vi "get Object By Name.vi"(10 "Name":string, 11 "Scene in":refnum<class "Scene.lvclass">) -> (2 "Index":i32, 3 "Object":T1)   [LabVIEW 2022 SP3, in "Application.lvlib" / "Scene.lvclass"]
uses:
  Scene.lvclass
  Libraries/3D/Object.ctl
  Libraries/3D/Triangle 3D.ctl
  Libraries/3D/Vector 3D.ctl
  Libraries/3D/Transform.ctl
  Scene.lvclass/Scene.ctl
  Libraries/3D/3D.lvlib
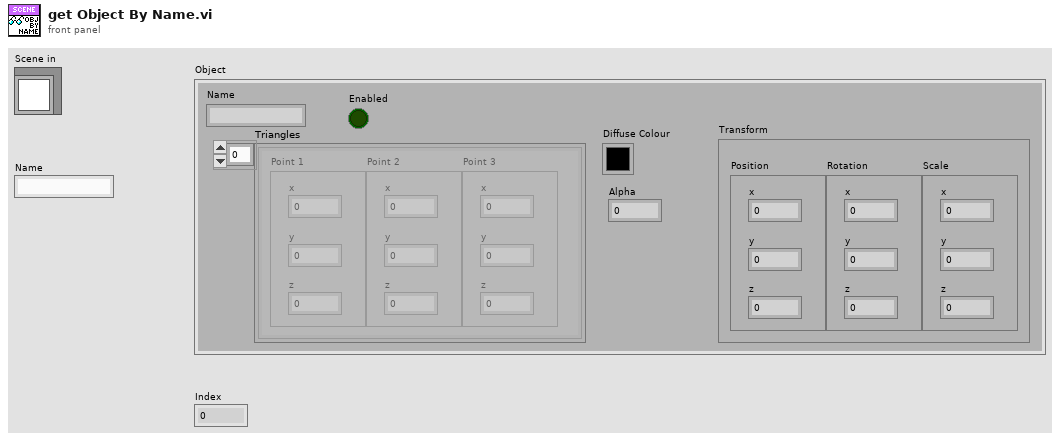
[diagram p1: front panel]
types:
  T1 = typedef "3D.lvlib/Object.ctl" = cluster{"Triangles":T2[], "Diffuse Colour":u32, "Transform":T4, "Name":string, "Enabled":bool, "Alpha":dbl}
  T2 = typedef "3D.lvlib/Triangle 3D.ctl" = cluster{"Point 1":T3, "Point 2":T3, "Point 3":T3}
  T3 = typedef "3D.lvlib/Vector 3D.ctl" = cluster{"x":sgl, "y":sgl, "z":sgl}
  T4 = typedef "3D.lvlib/Transform.ctl" = cluster{"Position":T3, "Rotation":T3, "Scale":T3}
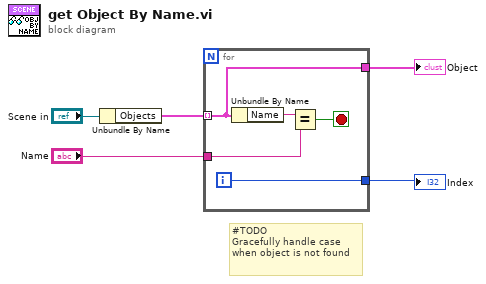
[diagram p0: block diagram]
diagram:
  # "#TODO\nGracefully handle case when object is not found"
  n1 = Unbundle By Name("Scene in") -> ("Objects"=w4:T1[])
  n2 = for {
    tunnel: w4 -> [w10] mode=indexing
    tunnel: [w10] -> w3
    tunnel: "Name" -> [w8]
    tunnel: [w6] -> w1
    i -> [w6]
    stop <- w7 stop-if-true
    n3 = Unbundle By Name(w10) -> ("Name"=w9:string)
    n4 = Equal?(x=w9, y=w8) -> (x = y?=w7:bool)
  }
  "Object" <- w3
  "Index" <- w1
